vi "Main.vi"   [LabVIEW 2018, in "Research.lvclass"]
uses:
  Research/Research.lvclass
  Person/Person.lvclass/Person.ctl
  Person/Person.lvclass
  Relationships/Relationships.lvclass
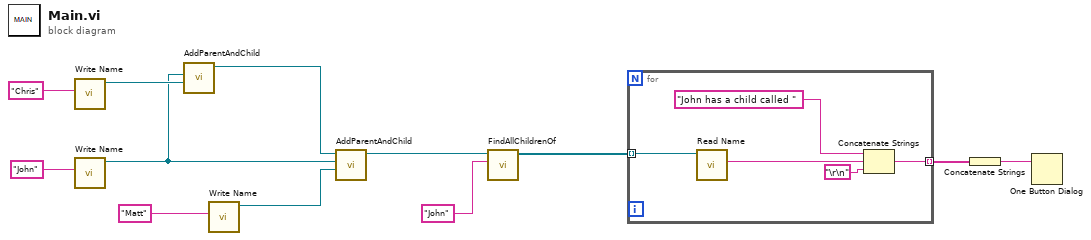
[diagram p0: block diagram]
diagram:
  n1 = call "Write Name.vi"("Name"="Chris") -> ("Person Out"=w9:refnum<class "Person.lvclass">)  [unwired: 10 in]
  n2 = call "Write Name.vi"("Name"="John") -> ("Person Out"=w8:refnum<class "Person.lvclass">)  [unwired: 10 in]
  n3 = call "AddParentAndChild.vi"("Child"=w9, "Parent"=w8) -> ("Relationships Out"=w6:refnum<class "Relationships.lvclass">)  [unwired: 9 in]
  n4 = call "Write Name.vi"("Name"="Matt") -> ("Person Out"=w7:refnum<class "Person.lvclass">)  [unwired: 10 in]
  n5 = call "AddParentAndChild.vi"("Child"=w7, "Parent"=w8, "Relationships In"=w6) -> ("Relationships Out"=w5:refnum<class "Relationships.lvclass">)  [unwired: 8 in]
  n6 = call-dynamic "FindAllChildrenOf.vi"("Name"="John", "RelationshipBrowser"=w5) -> ("Children"=w3:refnum<class "Person.lvclass">[])  [unwired: 9 in]
  n7 = for {
    tunnel: w3 -> [w17] mode=indexing
    tunnel: [w13] -> w2 mode=indexing
    n8 = call "Read Name.vi"("Person In"=w17) -> ("Name"=w15:string)  [unwired: 9 in, 1 out]
    n9 = Concatenate Strings("John has a child called " ("string"), w15, "\r\n") -> (w13:string)
  }
  n10 = Concatenate Strings(w2) -> (w1:string)
  n11 = One Button Dialog(message=w1) -> ()  [unwired: 1 in, 1 out]
